vi "Numeric to string to numeric.vi"() -> ()   [LabVIEW 2021]
panel:
  out "Int again":i32
  out "length 2":i32
  out "string 2":string
  in  "Int":i32
  out "Float again":dbl
  out "length":i32
  out "string":string
  in  "FLoat":dbl
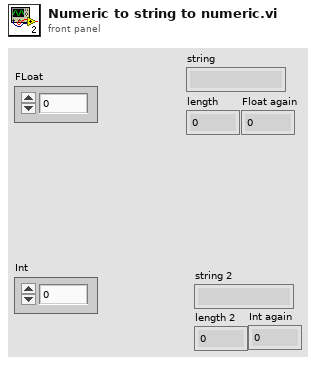
[diagram p1: front panel]
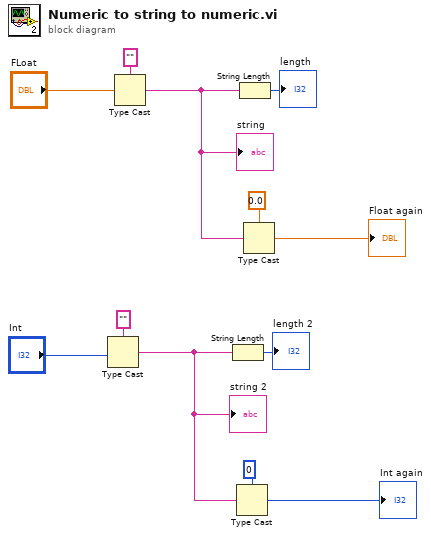
[diagram p0: block diagram]
diagram:
  n1 = Type Cast(type="", x="Int") -> (*(type *) &x=w4:string)
  "string 2" <- w4
  n2 = Type Cast(type="", x="FLoat") -> (*(type *) &x=w7:string)
  "string" <- w7
  n3 = String Length(string=w4) -> (length=→"length 2":i32)
  n4 = Type Cast(type=0, x=w4) -> (*(type *) &x=→"Int again":i32)
  n5 = String Length(string=w7) -> (length=→"length":i32)
  n6 = Type Cast(type=0.0, x=w7) -> (*(type *) &x=→"Float again":dbl)
